vi "CRYTest Input Param.vi"(11 "Flattend Analysis":string) -> (3 "test result":bool)   [LabVIEW 2013]
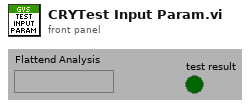
[diagram p1: front panel]
types:
  T1 = typedef "CRYAnalysis Cluster.ctl" = cluster{"Name":string, "Harmonics":dbl[], " Algorithm":u16, "delay":dbl, "THD(%)":bool, "Rub&Buzz":bool, "Imp":bool, "Imp Ref resistor":dbl, "Y data":u16, "Y prefix":string, "Y unit":string, "Y dB ref":dbl, "Custom Curve Names":string[], "har list items":string[], "Envelope":bool, "use custom unit":bool, "autodelay ch":dbl, "impulse":bool, " start ms":dbl, " stop ms":dbl, "Scaling":i32, "Default Overlap ":bool, "Advanced View":bool, "Loose Particle":bool, "Use default":bool, "Auto-Correlation(Stimulus)":bool, "Auto-Correlation(Response)":bool, "Deconvolved Response":bool, "Mic Current":bool, "M List Vaiues":u16, "Type":u16, "Delay Method":u16, "Apply Correction Out":bool, "Apply Correction In":bool, "Harmonics @ meas.frq":bool, "THD Normalized(%)":bool, "Total Distortion":bool, "THD+Noise(%)":bool, "Rub&Buzz Norm'd(%)":bool, "Standard Error":bool, "Confidence Limits":bool, "Total Diff":bool, "Total Noise":bool, "Total DFD(%)":bool, "Total IMD(%)":bool, "Total IM":bool, "Total DFD+Noise(%)":bool, "Use Channel Name":bool, "Waveform In":string, "Waveform Out":string, "Method":u16, "Spectral Scaling":u16, "Appliied Unit":u16, "Length Unit":u16, "Applied Units":u16, "Sens Item":u16, "Tab":i32, "Distance Unit":u16, "discard cycles":dbl, "Weigting":string, "Averaging Time":dbl, "Max duration":dbl, "Min duration":dbl, "Attack Threshold":dbl, "Hysteresis Up":dbl, "Fmin(Hz)":dbl, "Fmax(Hz)":dbl, "Freq.Resolution":dbl, "Over-samples Res.":dbl, "Win Resolution":dbl, "distance":dbl, "samples":dbl, "Overlap":dbl, "Record Length":dbl, "No.of FFTs":dbl, "Hz":dbl, "record delay":dbl, " Std Err":dbl, "Response":bool, "Coherent Power*":bool, "Stimulus":bool, "Measurement Confidence":bool, "Auto Spectrum(Response)*":bool, "Auto Spectrum(Stimulus)*":bool, "Cross Spectrum*":bool, "functions":bool, "Frequency Response":bool, "Non-Coherent Power*":bool, "Coherence (%)":bool, "Non-Coherence (%)":bool, "Signal-Noise Ratio (dB)":bool, "Non-Coherenct Distirtion*":bool, "Result Waveforms":bool, "Coupling":bool, "Averaging":u16, "Harmonics":i32, "Custom Curve Names":i32, "unLabel":string, "Custom Curve Names":string, "Unit":string, "Total IMD + Noise(%) ":bool, "ResponseMe":u16, "Intermod":dbl[], "Diff\n":dbl[], "Cross-Correlation":bool, "IM list items":string[], "Diff list items":string[], "TSR Window Type":string, "Help":string, "Custom Curve IDs":i32[], "Default Curve Names":string[], "Loose Particle waveform":bool, "Perceptual Rub&Buzz":bool, "Imp Auto Mode":u16, "Mic Auto Mode":u16, "Mic Ref resistor":dbl, "Curve Resolution":u16, "Curve Resolution Hz":dbl, "Polarity":bool}
  T2 = typedef "CRYWaveform Cluster.ctl" = cluster{"Waveform":cluster{"X0":dbl, "dX":dbl, "Y":sgl[]}, "X data":u16, "Y data":u16, "Y axis":u16, "X unit":string, "Y unit":string, "Y dB ref":dbl, "display Y":bool, "display X":bool, "Overload?":bool, "Test Info":string, "Step No.":i32, "Name":string, "protected":bool, "Sqc history":string[], "Signal Channel ID":i32, "Plot Settings":cluster{"Color":u32, "Interpolation":u8, "Point Style":u8, "Line Style":u8, "Point Color":u32, "Line Width":u8, "Bar Plot Style":u8, "Fill To":i16}, "AutoProtect":bool}
  T3 = typedef "CRYStimulus Test Infor Cluster.ctl" = cluster{"Stimulus Type":string, "Signal Type":string, "In/Out":bool, "FAPS":cluster{"freq":dbl, "ampl":dbl, "cycles":dbl, "samples":i32}[], "Sampling Rate":dbl, "Samples":i32, "Analysis Param":string, "Resolution":u16, "Steps":u32, "Analysis Value":dbl[], "Diff Freq":dbl, "FStart":dbl, "FStop":dbl, "Calibration Param":string, "Anti Alias":dbl, "Level Out1":dbl, "Level Out2":dbl, "EQ":bool}
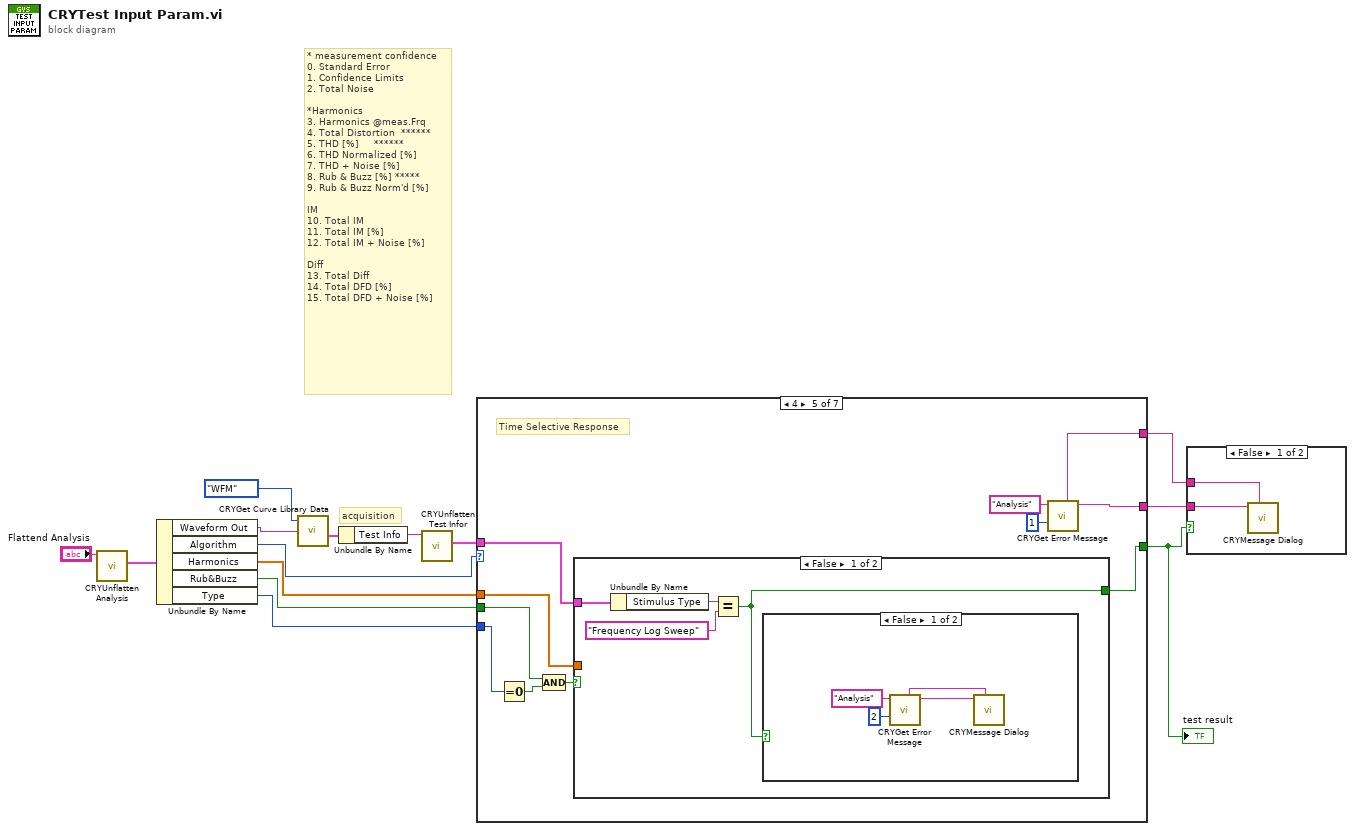
[diagram p0: block diagram]
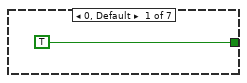
[diagram p2: hidden frame]
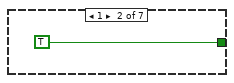
[diagram p3: hidden frame]
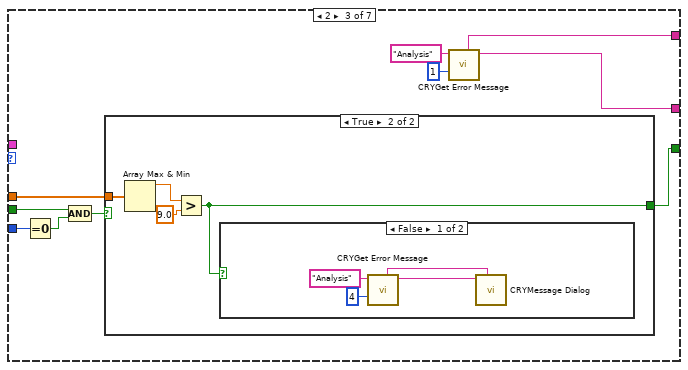
[diagram p4: hidden frame]
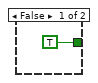
[diagram p5: hidden frame]
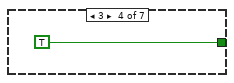
[diagram p7: hidden frame]
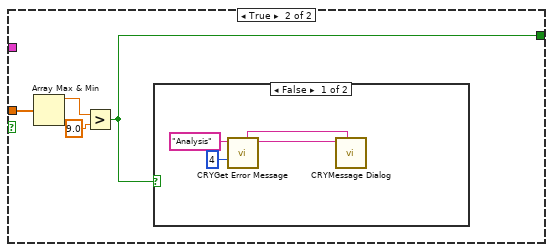
[diagram p9: hidden frame]
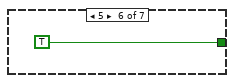
[diagram p11: hidden frame]
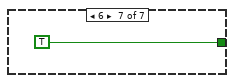
[diagram p12: hidden frame]
diagram:
  # "* measurement confidence\n0. Standard Error\n1. Confidence Limits\n2. Total Noise\n\n*Harmonics\n3. Harmonics @meas.Frq\n4. Total Distortion  ******\n5. THD [%]     ******\n6. THD Normalized [%]\n7. THD + Noise [%]\n8. Rub & Buzz [%] *****\n9. Rub & Buzz Norm'd [%]\n\nIM\n10. Total IM\n11. Total IM [%]\n12. Total IM + Noise [%]\n\nDiff\n13. Total Diff\n14. Total DFD [%]\n15. Total DFD + Noise [%]"
  # "acquisition"
  n1 = call "CRYUnflatten Analysis.vi"("Unflatten Analysis"="Flattend Analysis") -> ("Analysis"=w11:T1)  [unwired: 10 out]
  n2 = Unbundle By Name(w11) -> ("Waveform Out"=w13:string, "Algorithm"=w7:u16, "Harmonics"=w5:dbl[], "Rub&Buzz"=w4:bool, "Type"=w3:u16)
  n3 = call "CRYGet Curve Library Data.vi"("Type"=enum16{"Curves", "Values", "Results", "WFM"}."WFM", "Data Name"=w13) -> ("Wave"=w14:T2)  [unwired: 4 out]
  n4 = Unbundle By Name(w14) -> ("Test Info"=w12:string)
  n5 = call "CRYUnflatten Test Infor.vi"("Falattend test infor"=w12) -> ("unflattened test infor data"=w9:T3)  [unwired: 9 out]
  n6 = case shown="4" w7 {
    tunnel: w9 -> [_ _ _ _ w39 _ _]
    tunnel: [TRUE TRUE w17 TRUE w37 TRUE TRUE] -> w1
    tunnel: [_ _ w19 _ w45 _ _] -> w8
    tunnel: w5 -> [_ _ w26 _ w41 _ _]
    tunnel: w4 -> [_ _ w25 _ w43 _ _]
    tunnel: w3 -> [_ _ w24 _ w42 _ _]
    tunnel: [_ _ w18 _ w38 _ _] -> w2
    frame 0, Default {
    }
    frame 1 {
    }
    frame 2 {
      n7 = Equal To 0?(x=w24) -> (x = 0?=w23:bool)
      n8 = Compound Arithmetic op=AND(w25, w23) -> (w22:bool)
      n9 = case shown="True" w22 {
        tunnel: w26 -> [_ w31]
        tunnel: [TRUE w29] -> w17
        frame False {
        }
        frame True {
          n10 = Array Max & Min(array=w31) -> (max value=w28:dbl)  [unwired: 3 out]
          n11 = Greater?(x=w28, y=9.0) -> (0:w29:bool)
          n12 = case shown="False" w29 {
            frame False {
              n13 = call "CRYGet Error Message.vi"("Error No"=4, "Kind"="Analysis") -> ("Message"=w32:string, "Window Title"=w33:string)  [unwired: 4 in, 4 out]
              n14 = call "CRYMessage Dialog.vi"("Window Title"=w33, "Message Content"=w32) -> ()  [unwired: 8 in, 2 out]
            }
            frame True {
            }
          }
        }
      }
      n15 = call "CRYGet Error Message.vi"("Error No"=1, "Kind"="Analysis") -> ("Message"=w19:string, "Window Title"=w18:string)  [unwired: 4 in, 4 out]
    }
    frame 3 {
    }
    frame 4 {
      # "Time Selective Response"
      n16 = Equal To 0?(x=w42) -> (x = 0?=w44:bool)
      n17 = Compound Arithmetic op=AND(w43, w44) -> (w40:bool)
      n18 = case shown="False" w40 {
        tunnel: w41 -> [_ w59]
        tunnel: w39 -> [w49 _]
        tunnel: [w48 w56] -> w37
        frame False {
          n19 = Unbundle By Name(w49) -> ("Stimulus Type"=w50:string)
          n20 = Equal?(x=w50, y="Frequency Log Sweep") -> (x = y?=w48:bool)
          n21 = case shown="False" w48 {
            frame False {
              n22 = call "CRYGet Error Message.vi"("Error No"=2, "Kind"="Analysis") -> ("Message"=w52:string, "Window Title"=w53:string)  [unwired: 4 in, 4 out]
              n23 = call "CRYMessage Dialog.vi"("Window Title"=w53, "Message Content"=w52) -> ()  [unwired: 8 in, 2 out]
            }
            frame True {
            }
          }
        }
        frame True {
          n24 = Array Max & Min(array=w59) -> (max value=w57:dbl)  [unwired: 3 out]
          n25 = Greater?(x=w57, y=9.0) -> (0:w56:bool)
          n26 = case shown="False" w56 {
            frame False {
              n27 = call "CRYGet Error Message.vi"("Error No"=4, "Kind"="Analysis") -> ("Message"=w60:string, "Window Title"=w61:string)  [unwired: 4 in, 4 out]
              n28 = call "CRYMessage Dialog.vi"("Window Title"=w61, "Message Content"=w60) -> ()  [unwired: 8 in, 2 out]
            }
            frame True {
            }
          }
        }
      }
      n29 = call "CRYGet Error Message.vi"("Error No"=1, "Kind"="Analysis") -> ("Message"=w45:string, "Window Title"=w38:string)  [unwired: 4 in, 4 out]
    }
    frame 5 {
    }
    frame 6 {
    }
  }
  "test result" <- w1
  n30 = case shown="False" w1 {
    tunnel: w8 -> [w67 _]
    tunnel: w2 -> [w66 _]
    frame False {
      n31 = call "CRYMessage Dialog.vi"("Window Title"=w66, "Message Content"=w67) -> ()  [unwired: 8 in, 2 out]
    }
    frame True {
    }
  }
